vi "Lift.vi"   [LabVIEW 2018]
uses:
  <vilib>/Rock Robotics/SystemInterfaces/DIO/FPGA_DIOChannel.ctl
  <vilib>/Rock Robotics/WPI/ThirdParty/Phoenix-LabVIEW/Motor Controller/Controls/CTRE_Phoenix_MotorControl_ControlMode.ctl
  Lift Global.vi
  Times/Times Global.vi
  <vilib>/addons/control/pid/pid.llb/PID (DBL).vi
  <vilib>/Rock Robotics/WPI/ThirdParty/Phoenix-LabVIEW/Motor Controller/Get/CTRE_Phoenix_MotorController_GetSelectedSensorData.vi
  Cargo Intake/Cargo Intake Global.vi
  <vilib>/addons/control/pid/NI_PID_pid.lvlib
  <vilib>/Rock Robotics/WPI/Counter/WPI_CounterDigitalInputToDigitalSource.vi
types:
  T1 = typedef "FPGA_DIOChannel.ctl" = enum8{"DIO 0", "DIO 1", "DIO 2", "DIO 3", "DIO 4", "DIO 5", "DIO 6", "DIO 7", "DIO 8", "DIO 9", "DIO MXP 0", "DIO MXP 1", "DIO MXP 2", "DIO MXP 3", "DIO MXP 4", "DIO MXP 5", "DIO MXP 6", "DIO MXP 7", "DIO MXP 8", "DIO MXP 9", "DIO MXP 10", "DIO MXP 11", "DIO MXP 12", "DIO MXP 13", "DIO MXP 14", "DIO MXP 15", "SPI Port CS1", "SPI Port CS2", "SPI Port CS3", "SPI Port MISO", "SPI Port MOSI", "Invalid"}
  T2 = typedef "WPI_DigitalInputDevRef.ctl" = cluster{"DevStatus":errorcluster, "DIO Channel":T1}
  T3 = typedef "FPGA_CounterEncoderSourceConvertionLVSourceType.ctl" = cluster{"DevStatus":errorcluster, "AnalogTriggerMode?":bool, "DigitalMode":cluster{"DIO Channel":T4}, "AnalogTriggerMode":cluster{"AnalogTriggerIndex":T5, "OutputType":T6}}
  T4 = typedef "FPGA_DIODigitalSourceChannel.ctl" = enum8{"DIO 0", "DIO 1", "DIO 2", "DIO 3", "DIO 4", "DIO 5", "DIO 6", "DIO 7", "DIO 8", "DIO 9", "DIO MXP 0", "DIO MXP 1", "DIO MXP 2", "DIO MXP 3", "DIO MXP 4", "DIO MXP 5", "DIO MXP 6", "DIO MXP 7", "DIO MXP 8", "DIO MXP 9", "DIO MXP 10", "DIO MXP 11", "DIO MXP 12", "DIO MXP 13", "DIO MXP 14", "DIO MXP 15", "SPI Port CS1", "SPI Port CS2", "SPI Port CS3", "SPI Port MISO", "SPI Port MOSI", "Disabled"}
  T5 = typedef "FPGA_AnalogTriggerIndex.ctl" = enum8{"Trig 0", "Trig 1", "Trig 2", "Trig 3", "Trig 4", "Trig 5", "Trig 6", "Trig 7", "Invalid"}
  T6 = typedef "FPGA_AnalogTriggerOutType.ctl" = enum16{"InWindow", "TriggerState", "Rising", "Falling"}
  T7 = typedef "WPI_EncoderDevRef.ctl" = cluster{"DevStatus":errorcluster, "EncoderIndex":T8, "CounterIndex":T9, "DistancePerCount":dbl, "Decoding Type":T10}
  T8 = typedef "FPGA_EncoderIdx.ctl" = enum8{"Enc 0", "Enc 1", "Enc 2", "Enc 3", "Enc 4", "Enc 5", "Enc 6", "Enc 7", "Invalid"}
  T9 = typedef "FPGA_CounterCtrSystemIndex.ctl" = enum8{"Ctr 0", "Ctr 1", "Ctr 2", "Ctr 3", "Ctr 4", "Ctr 5", "Ctr 6", "Ctr 7", "Invalid"}
  T10 = typedef "WPI_EncoderType.ctl" = enum16{"1x", "2x", "4x"}
  T11 = enum16{"Ultra Manual Control", "Manual Control", "Basic Control", "Automated Control", "Autonomous Control"}
  T12 = enum16{"N/A", "Hatch Panel Zone 1", "Hatch Panel Zone 2", "Hatch Panel Zone 3", "Cargo Zone 1", "Cargo Zone 2", "Cargo Zone 3"}
  T13 = typedef "WPI_MotorControlDeviceRef.ctl" = cluster{"DeviceStatus":errorcluster, "Type":T14, "PWM":cluster{"PWM Channel":T15, "DeadBand":T16}, "CAN":cluster{"Device Number":u8, "SetOutput VI Ref":variant, "GetOutput VI Ref":variant, "Enable VI Ref":variant, "Disable VI Ref":variant, "Data":variant}, "Invert":bool, "DIO PWM":cluster{"PWM \"Enable\" Channel":T15, "DIOChannel":T1, "PWM Rate":dbl}}
  T14 = typedef "WPI_MotorControlType.ctl" = enum16{"PWM", "CAN", "DIO PWM"}
  T15 = typedef "FPGA_DIOPWMChannel.ctl" = enum8{"PWM 0", "PWM 1", "PWM 2", "PWM 3", "PWM 4", "PWM 5", "PWM 6", "PWM 7", "PWM 8", "PWM 9", "PWM MXP 0", "PWM MXP 1", "PWM MXP 2", "PWM MXP 3", "PWM MXP 4", "PWM MXP 5", "PWM MXP 6", "PWM MXP 7", "PWM MXP 8", "PWM MXP 9", "Invalid"}
  T16 = typedef "WPI_PWMDeadband.ctl" = cluster{"Name":string, "maxPositivePwm":i32, "minPositivePwm":i32, "centerPwm":i32, "maxNegativePwm":i32, "minNegativePwm":i32, "angularRange":u16}
  T17 = typedef "CTRE_Phoenix_MotorControl_ControlMode.ctl" = u16
  T18 = typedef "Control 3.ctl" = dbl
  T19 = cluster{"proportional gain (Kc)":dbl, "integral time(Ti, min)":dbl, "derivative time(Td, min) 2":dbl}
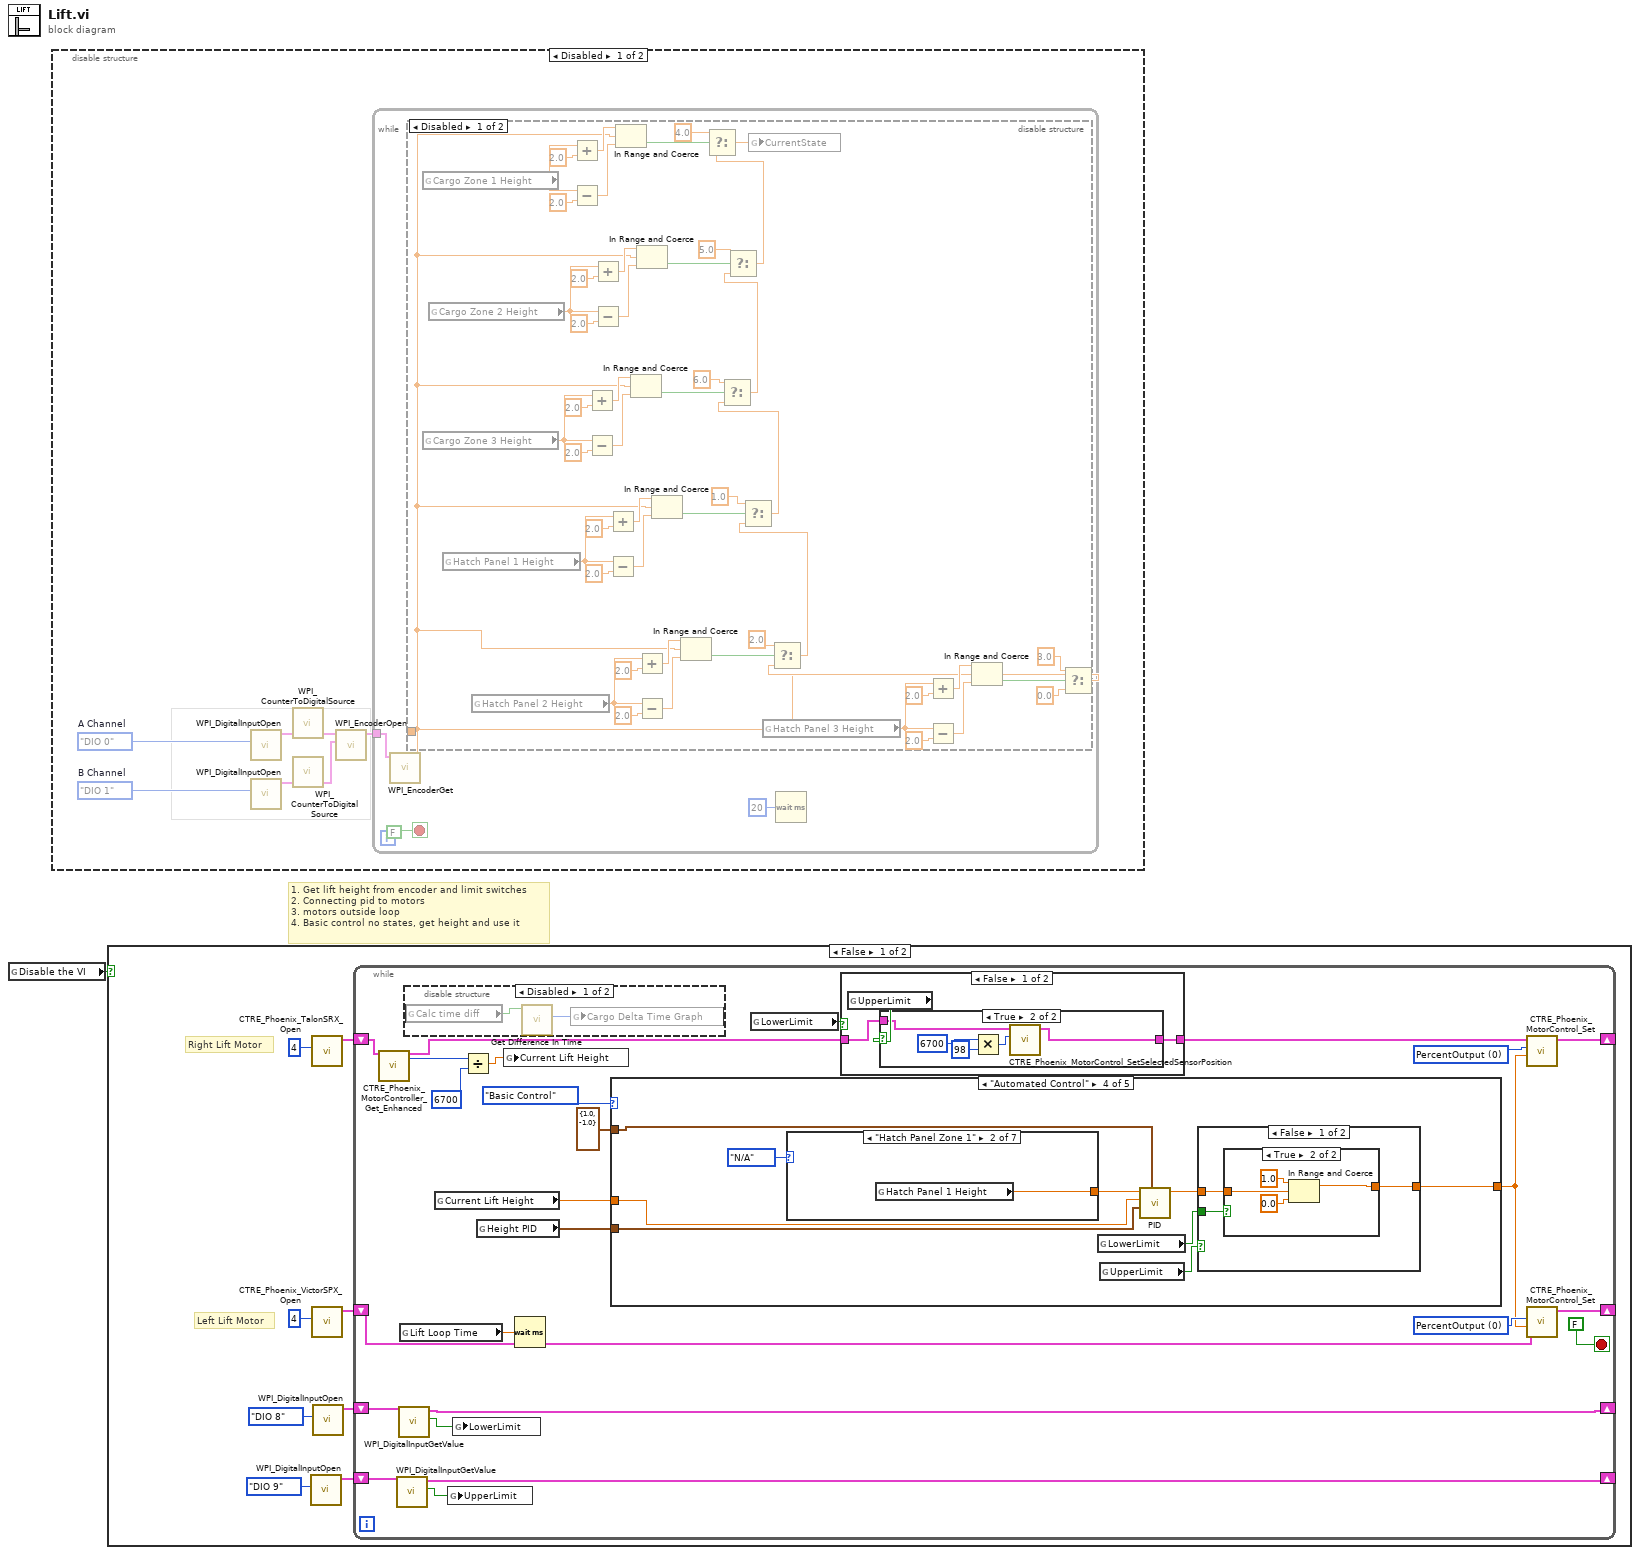
[diagram p0: block diagram]
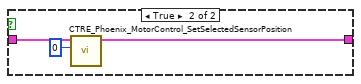
[diagram p5: hidden frame]
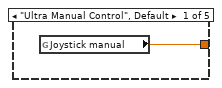
[diagram p7: hidden frame]
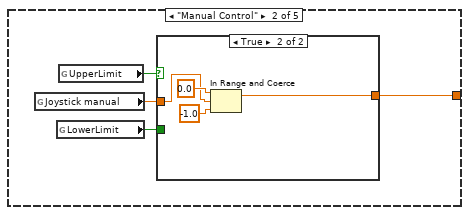
[diagram p8: hidden frame]
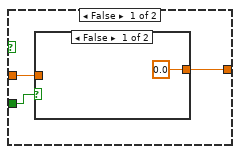
[diagram p9: hidden frame]
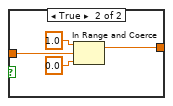
[diagram p10: hidden frame]
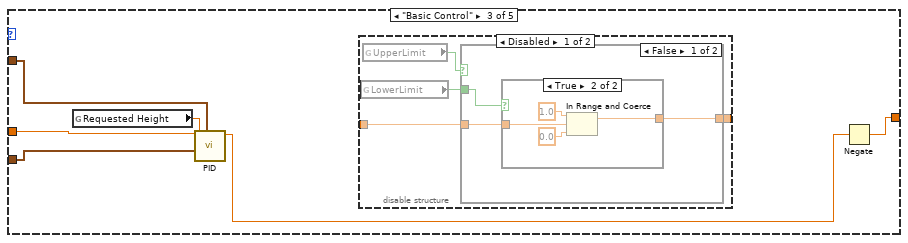
[diagram p11: hidden frame]
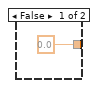
[diagram p12: hidden frame]
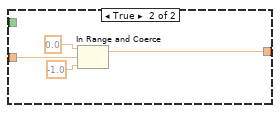
[diagram p13: hidden frame]
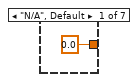
[diagram p15: hidden frame]
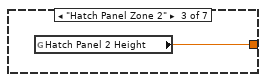
[diagram p16: hidden frame]
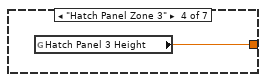
[diagram p17: hidden frame]
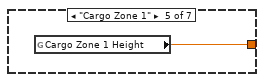
[diagram p18: hidden frame]
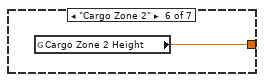
[diagram p19: hidden frame]
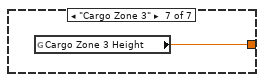
[diagram p20: hidden frame]
diagram:
  # "1. Get lift height from encoder and limit switches\n2. Connecting pid to motors\n3. motors outside loop\n4. Basic control no states, get height and use it"
  n1 = global read "Lift Global.vi" "Disable the VI"() -> (w1:bool)
  n2 = disable-structure shown="Disabled" {
    frame Disabled {
      w8 = FPGA_DIOChannel."DIO 1"  # B Channel
      w7 = FPGA_DIOChannel."DIO 0"  # A Channel
      n3 = call <vilib>:"WPI_DigitalInputOpen.vi"("DIO Channel"=w7) -> ("DigitalInputDevRef"=w4:T2)  [unwired: 1 in, 9 out]
      n4 = call <vilib>:"WPI_DigitalInputOpen.vi"("DIO Channel"=w8) -> ("DigitalInputDevRef"=w5:T2)  [unwired: 1 in, 9 out]
      n5 = call-poly <vilib>:"WPI_CounterToDigitalSource.vi"("DigitalInputDevRef"=w4) -> ("Digital Source"=w3:T3)  [unwired: 6 out]
      n6 = call-poly <vilib>:"WPI_CounterToDigitalSource.vi"("DigitalInputDevRef"=w5) -> ("Digital Source"=w6:T3)  [unwired: 6 out]
      n7 = call <vilib>:"WPI_EncoderOpen.vi"("BSource"=w6, "ASource"=w3) -> ("EncoderDevRef"=w2:T7)  [unwired: 6 in, 3 out]
      n8 = while {
        tunnel: w2 -> [w12]
        stop <- FALSE stop-if-true
        n9 = call <vilib>:"WPI_EncoderGet.vi"("EncoderDevRef"=w12) -> ("Distance"=w10:dbl)  [unwired: 5 in, 5 out]
        n10 = disable-structure shown="Disabled" {
          disable-tunnel: w10 -> [w13 _]
          frame Disabled {
            n11 = global read "Lift Global.vi" "Cargo Zone 1 Height"() -> (w53:dbl)
            n12 = global read "Lift Global.vi" "Cargo Zone 3 Height"() -> (w41:dbl)
            n13 = global read "Lift Global.vi" "Cargo Zone 2 Height"() -> (w59:dbl)
            n14 = global read "Lift Global.vi" "Hatch Panel 1 Height"() -> (w47:dbl)
            n15 = global read "Lift Global.vi" "Hatch Panel 2 Height"() -> (w29:dbl)
            n16 = Add(x=w53, y=2.0) -> (x+y=w55:dbl)
            n17 = Subtract(x=w53, y=2.0) -> (x-y=w56:dbl)
            n18 = Add(x=w41, y=2.0) -> (x+y=w43:dbl)
            n19 = Subtract(x=w41, y=2.0) -> (x-y=w44:dbl)
            n20 = Add(x=w59, y=2.0) -> (x+y=w61:dbl)
            n21 = Subtract(x=w59, y=2.0) -> (x-y=w62:dbl)
            n22 = Add(x=w47, y=2.0) -> (x+y=w49:dbl)
            n23 = Subtract(x=w47, y=2.0) -> (x-y=w50:dbl)
            n24 = In Range and Coerce(upper limit=w55, x=w13, lower limit=w56) -> (In Range?=w51:bool)  [unwired: 1 out]
            n25 = In Range and Coerce(upper limit=w43, x=w13, lower limit=w44) -> (In Range?=w39:bool)  [unwired: 1 out]
            n26 = In Range and Coerce(upper limit=w61, x=w13, lower limit=w62) -> (In Range?=w57:bool)  [unwired: 1 out]
            n27 = Add(x=w29, y=2.0) -> (x+y=w31:dbl)
            n28 = Subtract(x=w29, y=2.0) -> (x-y=w32:dbl)
            n29 = In Range and Coerce(upper limit=w49, x=w13, lower limit=w50) -> (In Range?=w45:bool)  [unwired: 1 out]
            n30 = In Range and Coerce(upper limit=w31, x=w13, lower limit=w32) -> (In Range?=w27:bool)  [unwired: 1 out]
            n31 = global read "Lift Global.vi" "Hatch Panel 3 Height"() -> (w35:dbl)
            n32 = Add(x=w35, y=2.0) -> (x+y=w37:dbl)
            n33 = Subtract(x=w35, y=2.0) -> (x-y=w38:dbl)
            n34 = In Range and Coerce(upper limit=w37, x=w13, lower limit=w38) -> (In Range?=w33:bool)  [unwired: 1 out]
            n35 = Select(t=3.0, s=w33, f=0.0 ("t")) -> (s? t:f=w23:dbl)
            n36 = Select(t=2.0, s=w27, f=w23) -> (s? t:f=w24:dbl)
            n37 = Select(t=1.0, s=w45, f=w24) -> (s? t:f=w25:dbl)
            n38 = Select(t=6.0, s=w39, f=w25) -> (s? t:f=w26:dbl)
            n39 = Select(t=5.0, s=w57, f=w26) -> (s? t:f=w20:dbl)
            n40 = Select(t=4.0, s=w51, f=w20) -> (s? t:f=w21:dbl)
            n41 = global write "Lift Global.vi" "CurrentState"(w21) -> ()
          }
          frame Enabled {
          }
        }
        n42 = Wait (ms)(milliseconds to wait=u32 20) -> ()  [unwired: 1 out]
      }
    }
    frame Enabled {
    }
  }
  n43 = case shown="False" w1 {
    frame False {
      # "Left Lift Motor"
      # "Right Lift Motor"
      n44 = call <vilib>:"WPI_DigitalInputOpen.vi"("DIO Channel"=FPGA_DIOChannel."DIO 9") -> ("DigitalInputDevRef"=w63:T2)  [unwired: 9 in, 1 out]
      n45 = call <vilib>:"CTRE_Phoenix_TalonSRX_Open.vi"("Device Number"=u8 4) -> ("CAN Talon SRX Ref"=w70:T13)  [unwired: 9 in, 1 out]
      n46 = call <vilib>:"CTRE_Phoenix_VictorSPX_Open.vi"("Device Number"=u8 4) -> ("CAN Talon SRX Ref"=w68:T13)  [unwired: 9 in, 1 out]
      n47 = call <vilib>:"WPI_DigitalInputOpen.vi"("DIO Channel"=FPGA_DIOChannel."DIO 8") -> ("DigitalInputDevRef"=w65:T2)  [unwired: 9 in, 1 out]
      n48 = while {
        shift-right: [w91] -> _
        shift-left: w70 -> [w83]
        shift-right: [w89] -> _
        shift-left: w68 -> [w88]
        shift-right: [w76] -> _
        shift-left: w65 -> [w77]
        shift-right: [w71] -> _
        shift-left: w63 -> [w72]
        stop <- FALSE stop-if-true
        w90 = T17 0 items=["PercentOutput"=0, "Position"=1, "Velocity"=2, "Current"=3, "Follower"=5, "MotionProfile"=6, "MotionMagic"=7, "MotionProfileArc"=10, "Disabled"=15] ("Control Mode")
        w92 = T17 0 items=["PercentOutput"=0, "Position"=1, "Velocity"=2, "Current"=3, "Follower"=5, "MotionProfile"=6, "MotionMagic"=7, "MotionProfileArc"=10, "Disabled"=15] ("Control Mode")
        n49 = call-poly <vilib>:"CTRE_Phoenix_MotorController_Get_Enhanced.vi"("PhoenixMotorControlDevRef"=w83) -> ("PhoenixMotorControlDevRef"=w82:T13, "Position (Raw Sensor Units)"=w80:i32)  [unwired: 11 in, 2 out]
        n50 = call <vilib>:"WPI_DigitalInputGetValue.vi"("DigitalInputDevRef"=w72) -> ("Value"=w74:bool, "DigitalInputDevRef"=w71:T2)  [unwired: 8 in, 1 out]
        n51 = call <vilib>:"WPI_DigitalInputGetValue.vi"("DigitalInputDevRef"=w77) -> ("Value"=w75:bool, "DigitalInputDevRef"=w76:T2)  [unwired: 8 in, 1 out]
        n52 = global read "Times Global.vi" "Lift Loop Time"() -> (w95:T18)
        n53 = disable-structure shown="Disabled" {
          frame Disabled {
            n54 = global read "Cargo Intake Global.vi" "Calc time diff"() -> (w109:bool)
            n55 = call "Get Difference In Time.vi"("Calculate Time Difference"=w109) -> ("Delta Time over Time"=w108:u32)  [unwired: 9 in, 1 out]
            n56 = global write "Times Global.vi" "Cargo Delta Time Graph"(w108) -> ()
          }
          frame Enabled {
          }
        }
        n57 = global read "Lift Global.vi" "Current Lift Height"() -> (w84:dbl)
        n58 = global write "Lift Global.vi" "UpperLimit"(w74) -> ()
        n59 = global write "Lift Global.vi" "LowerLimit"(w75) -> ()
        n60 = Divide(x=w80, y=6700) -> (x/y=w79:dbl)
        n61 = global read "Lift Global.vi" "Height PID"() -> (w85:T19)
        n62 = global write "Lift Global.vi" "Current Lift Height"(w79) -> ()
        n63 = Wait (ms)(milliseconds to wait=w95) -> ()  [unwired: 1 out]
        n64 = case shown="\"Automated Control\"" T11."Basic Control" ("LiftMode") {
          tunnel: [w110 w111 w128 w154 0.0 ("Cargo Zone 3 Height")] -> w87
          tunnel: w84 -> [_ _ w132 w152 _]
          tunnel: w85 -> [_ _ w131 w151 _]
          tunnel: cluster{"output high":dbl, "output low":dbl} {"output high"=1.0, "output low"=-1.0} ("output range") -> [_ _ w130 w153 _]
          frame "Ultra Manual Control", Default {
            n65 = global read "Lift Global.vi" "Joystick manual"() -> (w110:dbl)
          }
          frame "Manual Control" {
            n66 = global read "Lift Global.vi" "Joystick manual"() -> (w112:dbl)
            n67 = global read "Lift Global.vi" "LowerLimit"() -> (w114:bool)
            n68 = global read "Lift Global.vi" "UpperLimit"() -> (w113:bool)
            n69 = case shown="True" w113 {
              tunnel: w114 -> [w117 _]
              tunnel: [w116 w124] -> w111
              tunnel: w112 -> [w115 w123]
              frame False {
                n70 = case shown="False" w117 {
                  tunnel: [0.0 w122] -> w116
                  tunnel: w115 -> [_ w119]
                  frame False {
                  }
                  frame True {
                    n71 = In Range and Coerce(upper limit=1.0, x=w119, lower limit=0.0) -> (coerced(x)=w122:dbl)  [unwired: 1 out]
                  }
                }
              }
              frame True {
                n72 = In Range and Coerce(upper limit=0.0, x=w123, lower limit=-1.0) -> (coerced(x)=w124:dbl)  [unwired: 1 out]
              }
            }
          }
          frame "Basic Control" {
            n73 = global read "Lift Global.vi" "Requested Height"() -> (w129:dbl)
            n74 = call-poly <vilib>:"PID.vi"("output range"=w130, "PID gains"=w131, "process variable"=w132, "setpoint"=w129) -> ("output"=w127:dbl)  [unwired: 6 in, 1 out]
            n75 = disable-structure shown="Disabled" {
              disable-tunnel: _ -> [w134 _]
              disable-tunnel: [w133 _] -> _
              frame Disabled {
                n76 = global read "Lift Global.vi" "LowerLimit"() -> (w136:bool)
                n77 = global read "Lift Global.vi" "UpperLimit"() -> (w135:bool)
                n78 = case shown="False" w135 {
                  tunnel: w136 -> [w139 _]
                  tunnel: [w138 w146] -> w133
                  tunnel: w134 -> [w137 w145]
                  frame False {
                    n79 = case shown="True" w139 {
                      tunnel: [0.0 w144] -> w138
                      tunnel: w137 -> [_ w141]
                      frame False {
                      }
                      frame True {
                        n80 = In Range and Coerce(upper limit=1.0, x=w141, lower limit=0.0) -> (coerced(x)=w144:dbl)  [unwired: 1 out]
                      }
                    }
                  }
                  frame True {
                    n81 = In Range and Coerce(upper limit=0.0, x=w145, lower limit=-1.0) -> (coerced(x)=w146:dbl)  [unwired: 1 out]
                  }
                }
              }
              frame Enabled {
              }
            }
            n82 = Negate(x=w127) -> (-x=w128:dbl)
          }
          frame "Automated Control" {
            n83 = case shown="\"Hatch Panel Zone 1\"" T12."N/A" ("LiftLocation") {
              tunnel: [0.0 ("Cargo Zone 3 Height") w159 w160 w161 w162 w163 w164] -> w149
              frame "N/A", Default {
              }
              frame "Hatch Panel Zone 1" {
                n84 = global read "Lift Global.vi" "Hatch Panel 1 Height"() -> (w159:dbl)
              }
              frame "Hatch Panel Zone 2" {
                n85 = global read "Lift Global.vi" "Hatch Panel 2 Height"() -> (w160:dbl)
              }
              frame "Hatch Panel Zone 3" {
                n86 = global read "Lift Global.vi" "Hatch Panel 3 Height"() -> (w161:dbl)
              }
              frame "Cargo Zone 1" {
                n87 = global read "Lift Global.vi" "Cargo Zone 1 Height"() -> (w162:dbl)
              }
              frame "Cargo Zone 2" {
                n88 = global read "Lift Global.vi" "Cargo Zone 2 Height"() -> (w163:dbl)
              }
              frame "Cargo Zone 3" {
                n89 = global read "Lift Global.vi" "Cargo Zone 3 Height"() -> (w164:dbl)
              }
            }
            n90 = global read "Lift Global.vi" "LowerLimit"() -> (w157:bool)
            n91 = global read "Lift Global.vi" "UpperLimit"() -> (w156:bool)
            n92 = call-poly <vilib>:"PID.vi"("output range"=w153, "PID gains"=w151, "process variable"=w152, "setpoint"=w149) -> ("output"=w155:dbl)  [unwired: 6 in, 1 out]
            n93 = case shown="False" w156 {
              tunnel: w157 -> [w167 _]
              tunnel: [w166 w174] -> w154
              tunnel: w155 -> [w165 w173]
              frame False {
                n94 = case shown="True" w167 {
                  tunnel: [0.0 w172] -> w166
                  tunnel: w165 -> [_ w169]
                  frame False {
                  }
                  frame True {
                    n95 = In Range and Coerce(upper limit=1.0, x=w169, lower limit=0.0) -> (coerced(x)=w172:dbl)  [unwired: 1 out]
                  }
                }
              }
              frame True {
                n96 = In Range and Coerce(upper limit=0.0, x=w173, lower limit=-1.0) -> (coerced(x)=w174:dbl)  [unwired: 1 out]
              }
            }
          }
          frame "Autonomous Control" {
          }
        }
        n97 = global read "Lift Global.vi" "LowerLimit"() -> (w73:bool)
        n98 = case shown="False" w73 {
          tunnel: w82 -> [w98 w107]
          tunnel: [w97 w106] -> w81
          frame False {
            n99 = global read "Lift Global.vi" "UpperLimit"() -> (w96:bool)
            n100 = case shown="True" w96 {
              tunnel: w98 -> [w99 w104]
              tunnel: [w99 w103] -> w97
              frame False {
              }
              frame True {
                n101 = Multiply(x=6700 ("y"), y=98 ("New Sensor Position")) -> (x*y=w100:i32)
                n102 = call <vilib>:"CTRE_Phoenix_MotorControl_SetSelectedSensorPosition.vi"("New Sensor Position"=w100, "PhoenixMotorControlDevRef"=w104) -> ("PhoenixMotorControlDevRef"=w103:T13)  [unwired: 8 in, 1 out]
              }
            }
          }
          frame True {
            n103 = call <vilib>:"CTRE_Phoenix_MotorControl_SetSelectedSensorPosition.vi"("New Sensor Position"=0, "PhoenixMotorControlDevRef"=w107) -> ("PhoenixMotorControlDevRef"=w106:T13)  [unwired: 8 in, 1 out]
          }
        }
        n104 = call <vilib>:"CTRE_Phoenix_MotorControl_Set.vi"("Output"=w87, "Control Mode"=w92, "PhoenixMotorControlDevRef"=w81) -> ("PhoenixMotorControlDevRef"=w91:T13)  [unwired: 7 in, 1 out]
        n105 = call <vilib>:"CTRE_Phoenix_MotorControl_Set.vi"("Output"=w87, "Control Mode"=w90, "PhoenixMotorControlDevRef"=w88) -> ("PhoenixMotorControlDevRef"=w89:T13)  [unwired: 7 in, 1 out]
      }
    }
    frame True {
    }
  }
